vi "CIInit.vi"() -> (3 "Camera data (out)":variant)   [LabVIEW 2011]
uses:
  CameraConfig.ctl
  BeadTracker2.llb/GenericCameraConfigType.ctl
  mkCameraData.ctl
panel:
  in  "Camera data":T1={"Session"=refnum, "Settings"={"Gain [1-4]"=1.0, "Offset"=50, "Mode"=6, "ROIs"=[], "ROI Size"={"X"=0, "Y"=0}, "Number of buffers"=40, "Use hardware multiple-ROI?"=FALSE, "GenericCameraConfig"={"Framerate (Hz)"=0, "Exposure time (us)"=0, "Image size"={"Width"=0, "Height"=0}}}} {"Settings"."Offset" min=50}
  in  "Camera settings":T2={"Gain [1-4]"=1.0, "Offset"=0, "Mode"=6, "ROIs"=[], "ROI Size"={"X"=100, "Y"=100}, "Number of buffers"=40, "Use hardware multiple-ROI?"=FALSE, "GenericCameraConfig"={"Framerate (Hz)"=200, "Exposure time (us)"=5000, "Image size"={"Width"=1280, "Height"=1024}}}
  # "us"
  # "us"
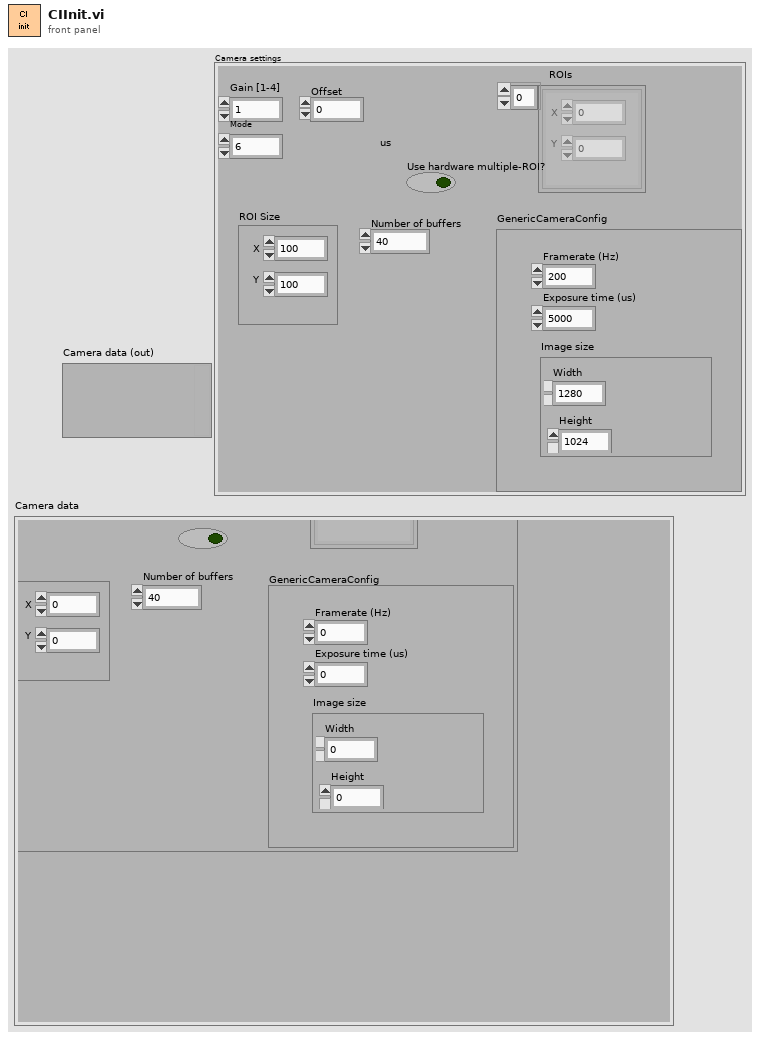
[diagram p1: front panel]
types:
  T1 = typedef "mkCameraData.ctl" = cluster{"Session":refnum<k11>, "Settings":T2}
  T2 = typedef "CameraConfig.ctl" = cluster{"Gain [1-4]":sgl, "Offset":i16, "Mode":i16, "ROIs":cluster{"X":i32, "Y":i32}[], "ROI Size":cluster{"X":i32, "Y":i32}, "Number of buffers":i32, "Use hardware multiple-ROI?":bool, "GenericCameraConfig":T3}
  T3 = typedef "GenericCameraConfigType.ctl" = cluster{"Framerate (Hz)":i32, "Exposure time (us)":i32, "Image size":cluster{"Width":i32, "Height":i32}}
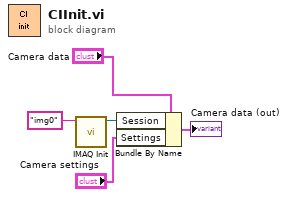
[diagram p0: block diagram]
diagram:
  n1 = call <vilib>:"IMAQ Init.vi"("Interface Name"="img0") -> ("IMAQ Session Out"=w3:refnum<k11>)  [unwired: 9 in, 1 out]
  n2 = Bundle By Name(cluster="Camera data", "Session"=w3, "Settings"="Camera settings") -> (→"Camera data (out)":T1)
